vi "Water_pressure_check.vi"(3 "error in":errorcluster, 4 "Step Number in":i32, 5 "Data in":T1) -> (0 "error out":errorcluster, 1 "Step Number out":i32, 2 "Data out":T1)   [LabVIEW 2015, in "Steps.lvlib"]
uses:
  Steps.lvlib
  Type_Defs/Data.ctl
  Type_Defs/Diagnostics.ctl
  Type_Defs/Systems.ctl
panel:
  in  "Step Back":bool
  in  "Continue":bool
  out "Water Pressure":dbl
  # "Options"
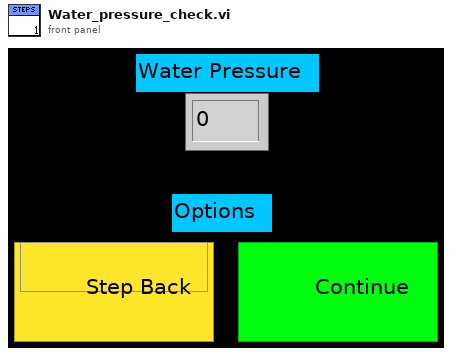
[diagram p1: front panel]
types:
  T1 = typedef "Data.ctl" = cluster{"User Name":string, "Experiment Number":i32, "Start Time":timestamp, "Data":dbl[], "Step Number":i32, "Step Instructions":string, "Diagnostics":T2, "Experiment Purpose":string, "Experiment State":enum16{"Off", "Setting Up", "Ready", "In Progress", "Shutting Down"}, "Systems":T3, "Current Pressure":dbl, "Fieldpoints":cluster{"System Boolean Fieldpoints":cluster{"Compressed Air":refnum<k21>, "T-20kV Power Switch":refnum<k21>, "T-Rectifier":refnum<k21>, "Engage Interlock":refnum<k21>, "Ventilator":refnum<k21>, "Magnetron":refnum<k21>, "H-20kV Power Switch":refnum<k21>, "H-Rectifier":refnum<k21>, "Main Water Pump":refnum<k21>, "WEGA Water Pump":refnum<k21>, "Gas Inlet Valves":refnum<k21>}, "Step Fieldpoints":cluster{"Exhaust Ventillator":refnum<k21>, "Compressed Air":refnum<k21>, "Water Pressure":refnum<k21>, "Interlock":refnum<k21>}}, "Pressure History":cluster{"Seconds into Experiement":i32[], "Pressure Data":dbl[]}}
  T2 = typedef "Diagnostics.ctl" = cluster{"Langmuir Probe":bool, "Rogowski 1":bool, "Rogowski 2":bool, "Rogowski 3":bool, "B-dot 1":bool, "B-dot 2":bool}
  T3 = typedef "Systems.ctl" = cluster{"Compressed Air":bool, "T-20kV Power Switch":bool, "T-Rectifier":bool, "Engage Interlock":bool, "Ventilator":bool, "Magnetron":bool, "H-20kV Power Switch":bool, "H-Rectifier":bool, "Main Water Pump":bool, "WEGA Water Pump":bool, "Gas Inlet Valves":bool}
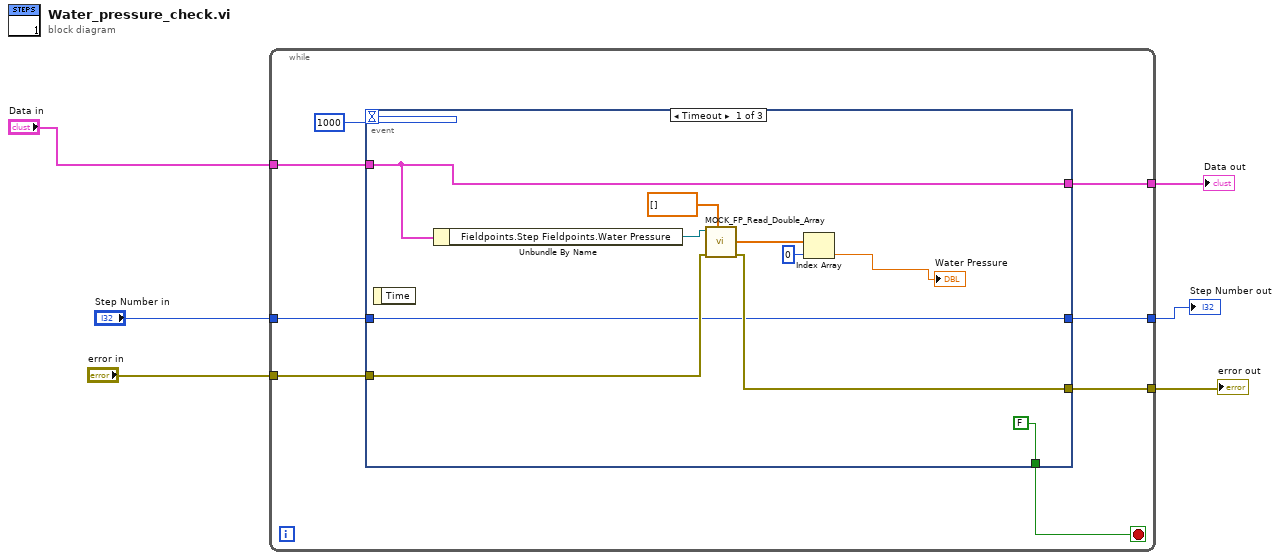
[diagram p0: block diagram]
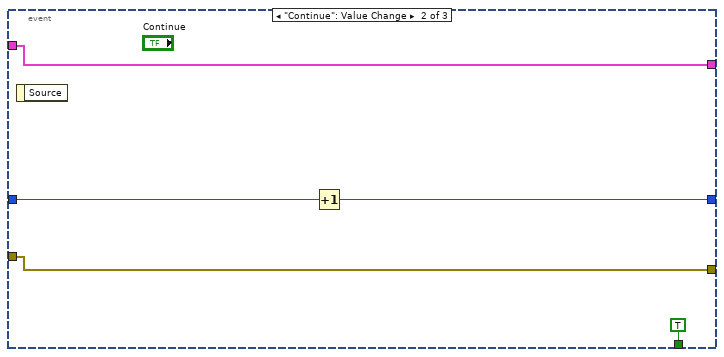
[diagram p2: hidden frame]
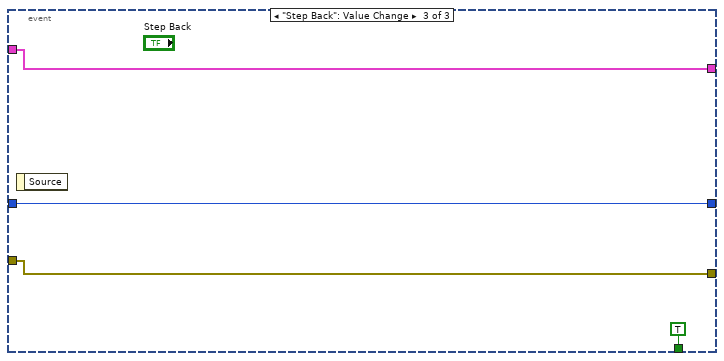
[diagram p3: hidden frame]
diagram:
  n1 = while {
    tunnel: "error in" -> [w13]
    tunnel: [w12] -> w2
    tunnel: [w10] -> w3
    tunnel: "Data in" -> [w9]
    tunnel: [w8] -> w5
    tunnel: "Step Number in" -> [w7]
    stop <- w11 stop-if-true
    n2 = event shown="[0] Timeout" {
      selector: _ -> [_ _ _]
      dyn-events: _ -> [_ _ _]
      timeout: 1000 -> [_ _ _]
      tunnel: w13 -> [w22 w28 w32]
      tunnel: [w21 w28 w32] -> w12
      tunnel: [FALSE TRUE TRUE] -> w11
      tunnel: [w19 w29 w33] -> w10
      tunnel: w9 -> [w19 w29 w33]
      tunnel: [w17 w26 w31] -> w8
      tunnel: w7 -> [w17 w27 w31]
      event Timeout {
        n3 = event-data() -> ()  [unwired: 1 in, 1 out]
        n4 = Unbundle By Name(w19) -> ("Fieldpoints.Step Fieldpoints.Water Pressure"=w18:refnum<k21>)
        n5 = call "MOCK_FP_Read_Double_Array.vi"("Type"=dbl[] [], "error in"=w22, "FieldPoint IO Point In"=w18) -> ("error out"=w21:errorcluster, "Array"=w24:dbl[])  [unwired: 5 in, 2 out]
        n6 = Index Array(array=w24, index=0) -> (element=→"Water Pressure":dbl)
      }
      event "Continue": Value Change {
        n7 = event-data() -> ()  [unwired: 1 in, 1 out]
        n8 = Increment(x=w27) -> (x+1=w26:i32)
      }
      event "Step Back": Value Change {
        n9 = event-data() -> ()  [unwired: 1 in, 1 out]
      }
    }
  }
  "error out" <- w2
  "Data out" <- w3
  "Step Number out" <- w5
